vi "Write GD Personal Log.vi"(8 "error in (no error)":errorcluster, 10 "String":string, 11 "Guardian in":refnum<class "Guardian.lvclass">) -> (0 "error out":errorcluster, 3 "Guardian out":refnum<class "Guardian.lvclass">)   [LabVIEW 2026, in "TALOS.lvlib" / "Guardian.lvlib" / "Guardian.lvclass"]
uses:
  Guardian.lvclass
  Guardian.lvclass/Guardian.ctl
  Classes/Log/Log.lvclass/Log.ctl
  Ancestor/Ancestor/Ancestor.lvclass/Ancestor.ctl
  Classes/Log/Write.vi
  Support VIs/Generate Error.vi
  Support VIs/Date n Time.vi
  FGV/Error Memory/Get Error Description.vi
  Support VIs/Get PC name.vi
  Ancestor/Ancestor/Read ID.vi
  Support VIs/Get Class Name.vi
  <vilib>/Utility/error.llb/Clear Errors.vi
  FGV/Error Memory/Error Memory Core.vi
  <vilib>/AdvancedString/Delimited String to 1D String Array.vi
  <vilib>/AdvancedString/Delimited String to 1D String Array (string).vi
  Support VIs/Circus Root Path.vi
  FGV/Error Memory/Error Crt Lvl checker.vi
  FGV/Error Memory/Error Memory Core.vi/40c8088d-b597-4017-91af-faa98e00292e.vi
  FGV/Error Memory/Error Memory Core.vi/d4a3ab98-063c-4e44-b43d-fbdcfe6c2be2.vi
  Classes/Log/Rotate.vi
  Support VIs/Global Memory.vi
  <vilib>/Utility/LVClass/Get LV Class Name.vi
  Support VIs/Is in Packed Library.vi
  Support VIs/TALOS Root path.vi
  Support VIs/Read CSV worksheet.vi
  Support VIs/Global Constants.vi
  <vilib>/Utility/error.llb/General Error Handler.vi
  Ancestor/Ancestor/Ancestor.lvclass
  <vilib>/Comparison/Equal/Equal Functor/Equal Functor.lvclass
  Classes/Log/Log.lvclass
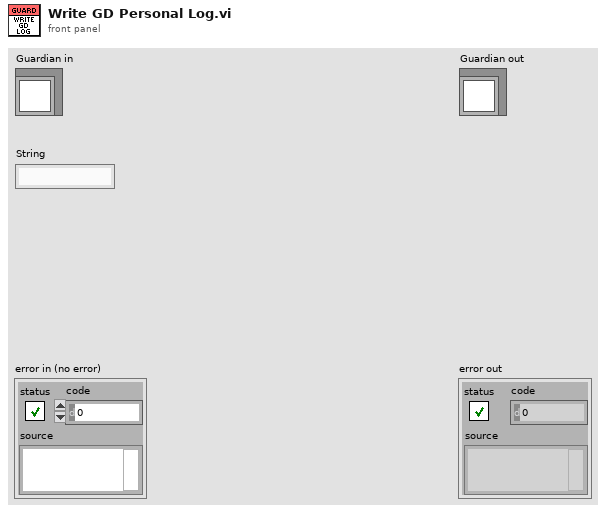
[diagram p1: front panel]
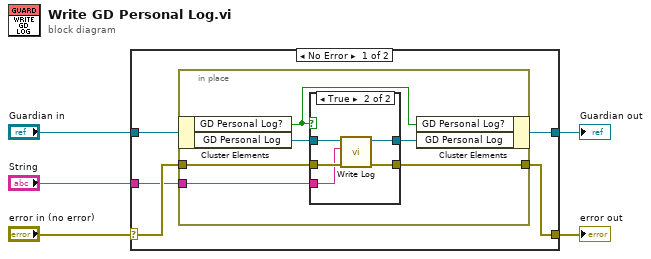
[diagram p0: block diagram]
diagram:
  n1 = case shown="No Error" "error in (no error)" {
    selector: "error in (no error)" -> [w8 w25]
    tunnel: [w7 w25] -> w4
    tunnel: [w9 w24] -> w2
    tunnel: "Guardian in" -> [w10 w24]
    tunnel: "String" -> [w6 _]
    frame No Error {
      n2 = in-place {
        in-place-border: w8 -> [w14]
        in-place-border: [w13] -> w7
        in-place-border: w6 -> [w12]
        n3 = in-place-cluster #1(w10) -> ("GD Personal Log?"=w11:bool, "GD Personal Log"=w16:refnum<class "Log.lvclass">)
        n4 = case shown="True" w11 {
          tunnel: w16 -> [w18 w23]
          tunnel: [w18 w22] -> w15
          tunnel: w14 -> [w17 w21]
          tunnel: [w17 w20] -> w13
          tunnel: w12 -> [_ w19]
          frame False {
          }
          frame True {
            n5 = call "Write Log.vi"("error in (no error)"=w21, "Text"=w19, "Log in"=w23) -> ("error out"=w20:errorcluster, "Log out"=w22:refnum<class "Log.lvclass">)  [unwired: 7 in]
          }
        }
        n6 = in-place-cluster #1("GD Personal Log?"=w11, "GD Personal Log"=w15) -> (w9:refnum<class "Guardian.lvclass">)
      }
    }
    frame Error {
    }
  }
  "error out" <- w4
  "Guardian out" <- w2
